vi "Analyze all images png.vi"() -> ()   [LabVIEW 2020]
uses:
  threshold ctl.ctl
  <userlib>/_MGI/File/Spreadsheet/MGI Write Spreadsheet Behavior Enum.ctl
  <vilib>/vision/NI_Vision_Development_Module.lvlib
panel:
  in  "Threshold":T1={"Use threshold fraction"=TRUE, "threshold fraction"=0.8, "Threshold Range"={"Lower value"=128.0, "Upper value"=255.0}}
  in  "Filename prefix":string
  in  "Tab Control":enum32{"Page 1", "Page 2"}(tab)
  in  "display":bool
  out "Numeric":i32
  out "subarray":string[](array[string])
  in  "index":i32
  in  "length":i32=2000
  out "Waveform Graph":sgl[](graph)
  out "Image":T2(plugin-control)
  in  "path":path=path "N:/data/Y2024/11-Nov/24_1107/analysis/kHzGhost/5_06_25 PM"
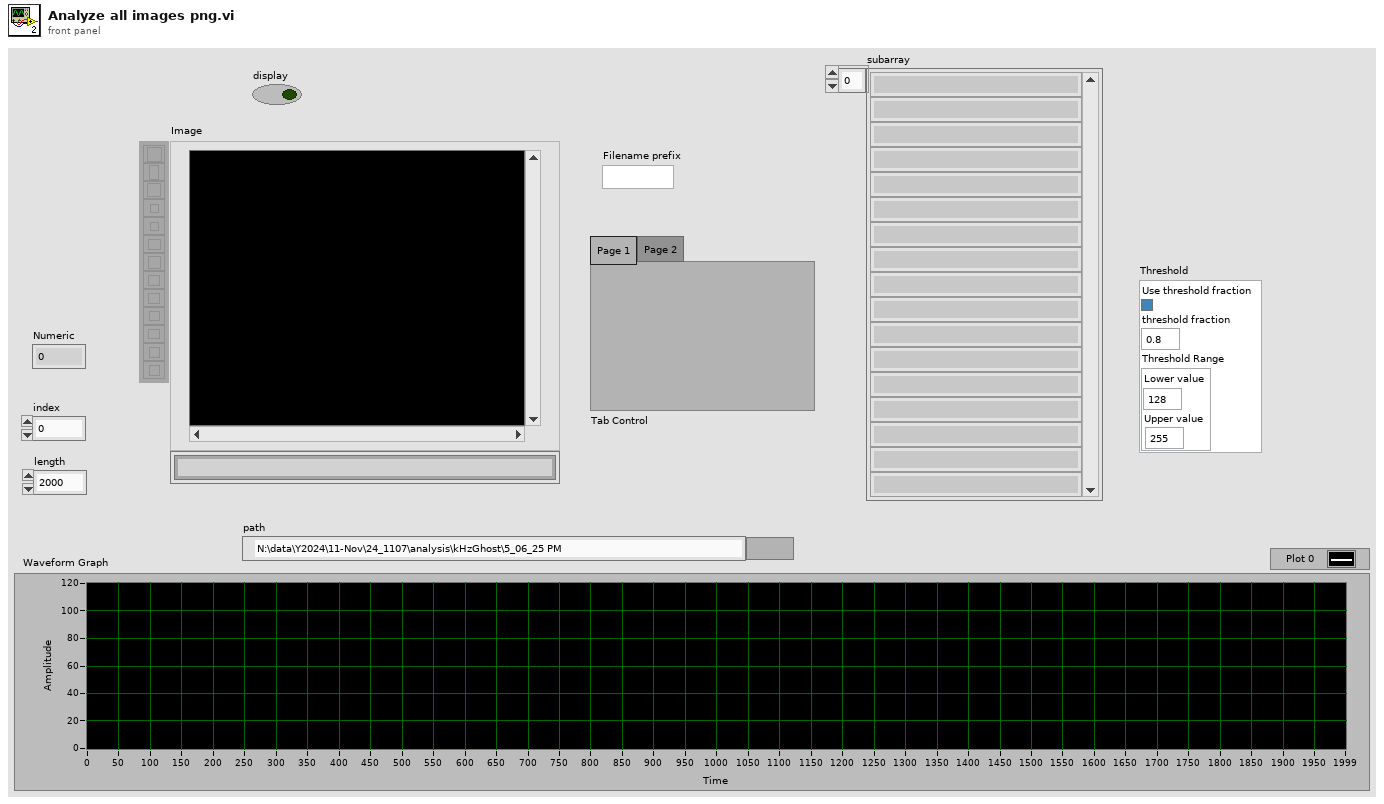
[diagram p1: front panel]
types:
  T1 = typedef "threshold ctl.ctl" = cluster{"Use threshold fraction":bool, "threshold fraction":sgl, "Threshold Range":cluster{"Lower value":sgl, "Upper value":sgl}}
  T2 = typedef "IMAQ Image.ctl" = refnum<image>
  T3 = typedef "MGI Write Spreadsheet Behavior Enum.ctl" = enum16{"Append data", "Append headers and data", "Overwrite"}
  T4 = typedef "Image Type" = u32
  T5 = cluster{"histogram":u32[], "Minimal Value":sgl, "Maximal Value":sgl, "Starting Value":sgl, "Interval Width":sgl, "Mean Value":sgl, "Standard  Variation":sgl, "Area (pixels)":i32}
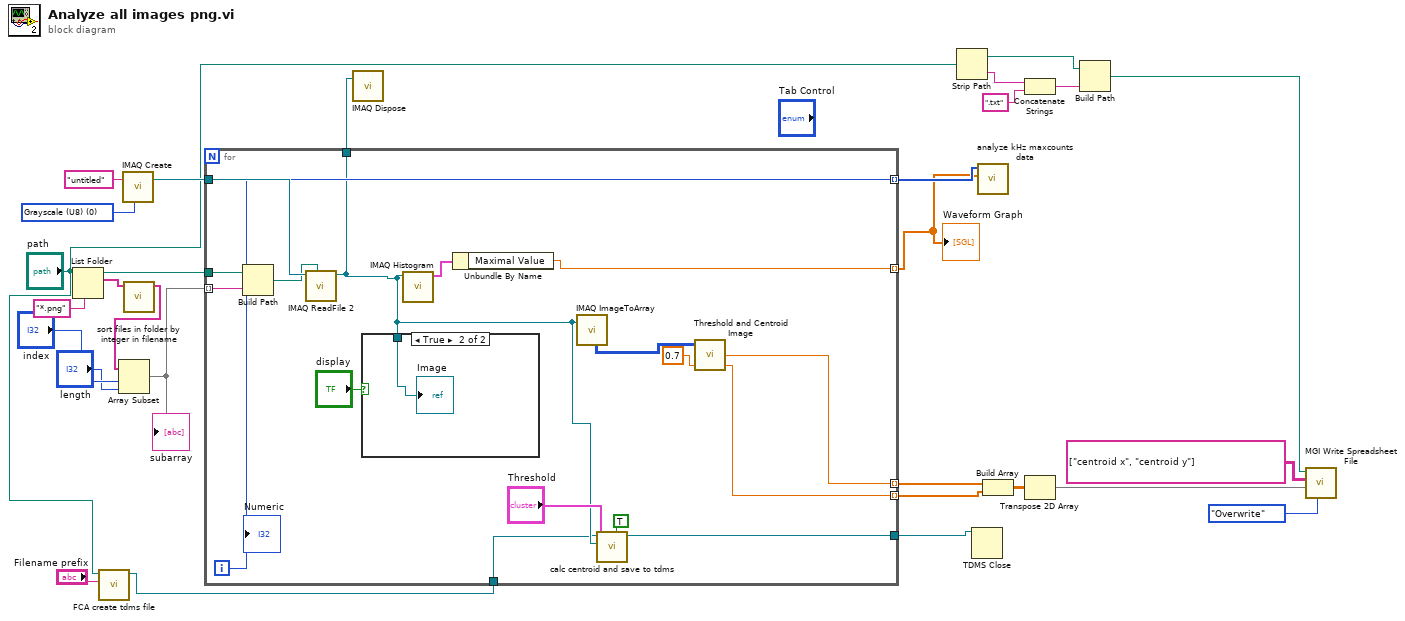
[diagram p0: block diagram]
diagram:
  w27 = T4 0 items=["Grayscale (U8)", "Grayscale (I16)", "Grayscale (SGL)", "Complex (CSG)", "RGB (U32)", "HSL (U32)", "RGB (U64)", "Grayscale (U16)"] ("Image Type")
  n1 = List Folder(path="path", pattern="*.png") -> (path out=w28:path, filenames=w18:string[])  [unwired: 2 in, 2 out]
  n2 = call "FCA create tdms file.vi"("Filename prefix"="Filename prefix", "Folder path"="path") -> ("Refnum out"=w3:refnum<k34>)  [unwired: 8 in, 1 out]
  n3 = call "IMAQ Create"("Image Name"="untitled", "Image Type"=w27) -> ("New Image"=w26:T2)  [unwired: 3 in, 1 out]
  n4 = call "sort files in folder by integer in filename.vi"("subarray"=w18) -> ("elements"=w17:string[])  [unwired: 10 in]
  n5 = Array Subset(array=w17, index="index", length="length") -> (w16:string[])
  "subarray" <- w16
  n6 = for {
    tunnel: w28 -> [w45]
    tunnel: w16 -> [w44] mode=indexing
    tunnel: w26 -> [w43]
    tunnel: [w31] -> w25
    tunnel: [w40] -> w19 mode=indexing
    tunnel: [w38] -> w20 mode=indexing
    tunnel: [w35] -> w11 mode=indexing
    tunnel: [w34] -> w10 mode=indexing
    tunnel: w3 -> [w30]
    tunnel: [w29] -> w2
    i -> [w38]
    n7 = Build Path(base path=w45, name or relative path=w44) -> (appended path=w42:path)
    n8 = call "IMAQ ReadFile 2"("File Path"=w42, "Image"=w43) -> ("Image Out"=w31:T2)  [unwired: 5 in, 4 out]
    n9 = case shown="True" "display" {
      tunnel: w31 -> [_ w46]
      frame False {
      }
      frame True {
        "Image" <- w46
      }
    }
    n10 = call "IMAQ Histogram"("Image"=w31) -> ("Histogram Report"=w41:T5)  [unwired: 9 in, 1 out]
    n11 = Unbundle By Name(w41) -> ("Maximal Value"=w40:sgl)
    n12 = call "IMAQ ImageToArray"("Image"=w31) -> ("Image Pixels (U16)"=w36:u16[][])  [unwired: 3 in, 4 out]
    n13 = call "calc centroid and save to tdms.vi"("tdms"=TRUE, "Threshold"="Threshold", "Image Out"=w31, "Refnum in"=w30) -> ("Refnum out"=w29:refnum<k34>)  [unwired: 5 in, 2 out]
    n14 = call "Threshold and Centroid Image.vi"("Raw Image"=w36, "Threshold or Threshold Fraction*"=0.7) -> ("x0"=w35:dbl, "y0"=w34:dbl)  [unwired: 2 in, 4 out]
    "Numeric" <- w38
  }
  "Waveform Graph" <- w19
  n15 = call "IMAQ Dispose"("Image"=w25) -> ()  [unwired: 5 in, 1 out]
  n16 = Strip Path(path="path") -> (stripped path=w6:path, name=w9:string)
  n17 = TDMS Close(11:w2) -> ()  [unwired: 1 in, 2 out]
  n18 = call "analyze kHz maxcounts data.vi"("Waveform Graph 3"=w19, "ramp"=w20) -> ()  [unwired: 10 in]
  n19 = Build Array(w11, w10) -> (w15:dbl[][])
  n20 = Concatenate Strings(w9, ".txt" ("string")) -> (w7:string)
  n21 = Transpose 2D Array(2D array=w15) -> (transposed array=w12:dbl[][])
  n22 = Build Path(base path=w6, name or relative path=w7) -> (appended path=w5:path)
  n23 = call <userlib>:"MGI Write Spreadsheet File.vi"("Existing File Behavior"=MGI_Write_Spreadsheet_Behavior_Enum."Overwrite", "Data[row][col]"=w12, "Header Lines[row][col]"=string[][] [["centroid x", "centroid y"]], "Path"=w5) -> ()  [unwired: 4 in, 4 out]
